vi "VCS Get Position Regulator Gain.vi"(8 "error in (no error)":errorcluster, 11 "axis in":cluster{"keyHandle":u32, "nodeId":u16}={"keyHandle"=0, "nodeId"=1}) -> (0 "error out":errorcluster, 2 "gains":T1, 3 "axis out":cluster{"keyHandle":u32, "nodeId":u16}={"keyHandle"=0, "nodeId"=1})   [LabVIEW 2019, in "maxonEPOS.lvlib"]
doc: "<B>VCS Get Position Regulator Gain</B> reads all position regulator gains."
uses:
  Examples/maxonEPOS.lvlib
  Resources/EposCmd.dll
  Resources/EposCmd64.dll
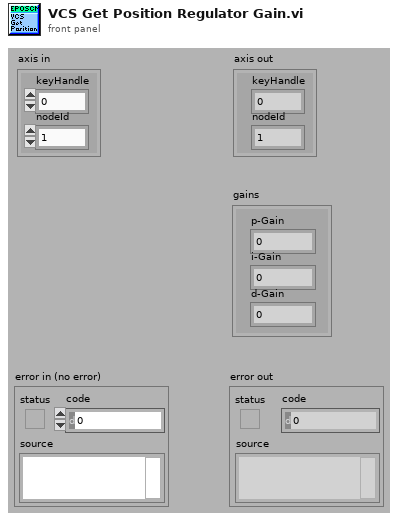
[diagram p1: front panel]
types:
  T1 = cluster{"p-Gain":u16, "i-Gain":u16, "d-Gain":u16}
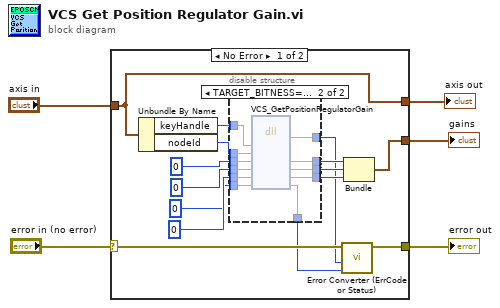
[diagram p0: block diagram]
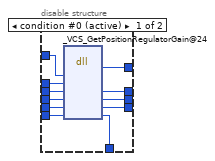
[diagram p2: hidden frame]
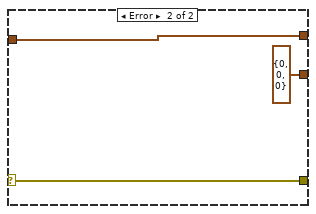
[diagram p3: hidden frame]
diagram:
  n1 = case shown="No Error" "error in (no error)" {
    selector: "error in (no error)" -> [w20 w45]
    tunnel: [w19 w45] -> w4
    tunnel: "axis in" -> [w7 w44]
    tunnel: [w8 cluster{"pP":u16, "pI":u16, "pD":u16} {"pP"=0, "pI"=0, "pD"=0}] -> w2
    tunnel: [w7 w44] -> w1
    frame No Error {
      n2 = Unbundle By Name(w7) -> ("keyHandle"=w17:u32, "nodeId"=w16:u16)
      n3 = disable-structure shown="TARGET_BITNESS==64" {
        disable-tunnel: [w31 w42] -> w18
        disable-tunnel: w17 -> [w30 w41]
        disable-tunnel: w16 -> [w29 w40]
        disable-tunnel: u16 0 ("pP") -> [w28 w39]
        disable-tunnel: u16 0 ("pI") -> [w27 w38]
        disable-tunnel: u16 0 ("pD") -> [w26 w37]
        disable-tunnel: u32 0 ("pErrorCode") -> [w25 w36]
        disable-tunnel: [w24 w35] -> w11
        disable-tunnel: [w23 w34] -> w10
        disable-tunnel: [w22 w33] -> w9
        disable-tunnel: [w21 w32] -> w6
        frame condition #0 (active) {
          n4 = dll-call lib="C:/workspace/project/scancon/sw/SSI_Tool/InstrumentsInterfaces/Motordriver/maxon EPOS/Resources/EposCmd.*" fn="_VCS_GetPositionRegulatorGain@24"("KeyHandle"=w30, "NodeId"=w29, "pP"=w28, "pI"=w27, "pD"=w26, "pErrorCode"=w25) -> (w21:i32, "pP"=w24:u16, "pI"=w23:u16, "pD"=w22:u16, "pErrorCode"=w31:u32)  [unwired: 5 in, 2 out]
        }
        frame condition #1 {
          n5 = dll-call lib="C:/Sources/LabView/maxon EPOS/Resources/EposCmd64.*" fn="VCS_GetPositionRegulatorGain" ("EposCmd.dll:_VCS_GetPositionRegulatorGain@24")("KeyHandle"=w41, "NodeId"=w40, "pP"=w39, "pI"=w38, "pD"=w37, "pErrorCode"=w36) -> ("Rückgabetyp"=w32:i32, "pP"=w35:u16, "pI"=w34:u16, "pD"=w33:u16, "pErrorCode"=w42:u32)  [unwired: 5 in, 2 out]
        }
      }
      n6 = call "Error Converter (ErrCode or Status).vi"("error code"=w18, "return type"=w6, "error in (no error)"=w20) -> ("error out"=w19:errorcluster)  [unwired: 7 in]
      n7 = Bundle("pP"=w11, "pI"=w10, "pD"=w9) -> (w8:cluster{"pP":u16, "pI":u16, "pD":u16})  [unwired: 1 in]
    }
    frame Error {
    }
  }
  "error out" <- w4
  "axis out" <- w1
  "gains" <- w2
